vi "Read ParsedData.vi"(8 "error in (no error)":errorcluster, 11 "CommandReceived in":refnum<class "CommandReceived.lvclass">) -> (0 "error out":errorcluster, 2 "ParsedData":refnum<class "ParsedData.lvclass">, 3 "CommandReceived out":refnum<class "CommandReceived.lvclass">)   [LabVIEW 2022 SP3, in "Cli.lvlib" / "CommandReceived.lvclass"]
uses:
  CommandReceived.lvclass
  CommandReceived.lvclass/CommandReceived.ctl
  ArgumentParser/Source/ParsedData/ParsedData.lvclass
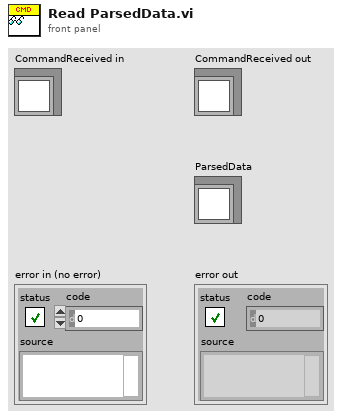
[diagram p1: front panel]
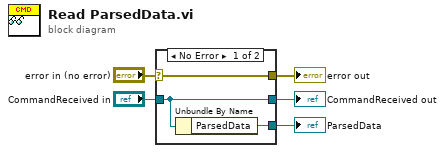
[diagram p0: block diagram]
diagram:
  n1 = case shown="No Error" "error in (no error)" {
    selector: "error in (no error)" -> [w8 w9]
    tunnel: [w8 w9] -> w4
    tunnel: [w7 w10] -> w2
    tunnel: "CommandReceived in" -> [w7 w10]
    tunnel: [w6 _] -> w1
    frame No Error {
      n2 = Unbundle By Name(w7) -> ("ParsedData"=w6:refnum<class "ParsedData.lvclass">)
    }
    frame Error {
    }
  }
  "error out" <- w4
  "CommandReceived out" <- w2
  "ParsedData" <- w1
